vi "AutoBalance.vi"(8 "error in (no error)":errorcluster) -> (0 "error out":errorcluster)   [LabVIEW 2023]
doc: "Wrapper class for drive straight"
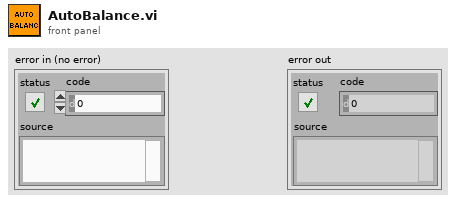
[diagram p1: front panel]
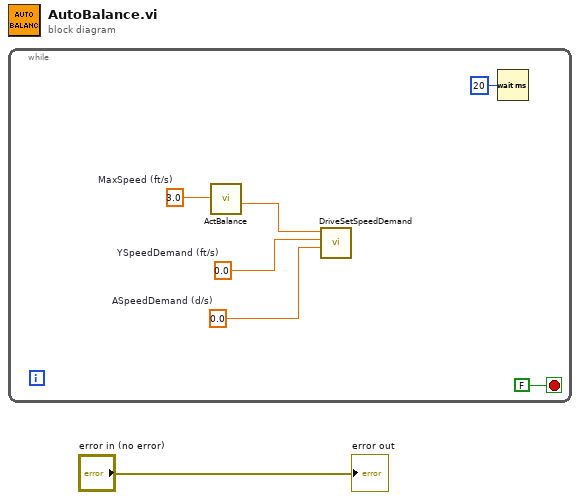
[diagram p0: block diagram]
diagram:
  n1 = while {
    stop <- FALSE stop-if-true
    w2 = 0.0  # ASpeedDemand (d/s)
    w3 = 0.0  # YSpeedDemand (ft/s)
    w4 = 3.0  # MaxSpeed (ft/s)
    n2 = call "ActBalance.vi"("MaxSpeed (ft/s)"=w4) -> ("XSpeedDemand"=w5:dbl)  [unwired: 9 in, 1 out]
    n3 = call "DriveSetSpeedDemand.vi"("ASpeedDemand (d/s)"=w2, "YSpeedDemand (ft/s)"=w3, "XSpeedDemand (ft/s)"=w5) -> ()  [unwired: 9 in]
    n4 = Wait (ms)(milliseconds to wait=u32 20) -> ()  [unwired: 1 out]
  }
  "error out" <- "error in (no error)"
